vi "实验3 频率调制RX.vi"() -> ()   [LabVIEW 2015]
uses:
  <vilib>/sound2/lvsound2.llb/Sound Data Format.ctl
  <instrlib>/niUSRP/niUSRP Fetch Rx Data (CDB WDT).vi
  <vilib>/sound2/lvsound2.llb/Sound Output Write (DBL Single).vi
  <vilib>/measure/maspectr.llb/FFT Power Spectrum and PSD for 1 Chan.vi
  <vilib>/measure/NI_MAPro.lvlib
panel:
  in  "采样点数":i64=20000
  in  "天线":string(combo)="RX2"
  in  "载波频率":dbl=800000000.0 format="%#_6p"
  in  "IQ 速率":dbl=400000.0 format="%#_6p"
  in  "增益":dbl format="%#_6f"
  in  "设备IP地址":refnum<k15>="192.168.10.2"
  in  "停止":bool
  out "FM解调时域信号":waveform(dbl)(graph)={"t0"=timestamp(3578355837.194731 s since 1904-01-01), "dt"=5.000000015582913e-06, "Y"=[]}
  out "FM解调频域信号":cluster{"f0":dbl, "df":dbl, "magnitude":dbl[]}(graph)={"f0"=0.0, "df"=9.999999968834175, "magnitude"=[]}
  in  "声音格式":T1={"sample rate (S/s)"=44100.0, "number of channels"=2, "bits per sample"=16}
  # "实验3 频率调制 RX"
  # "硬件参数配置"
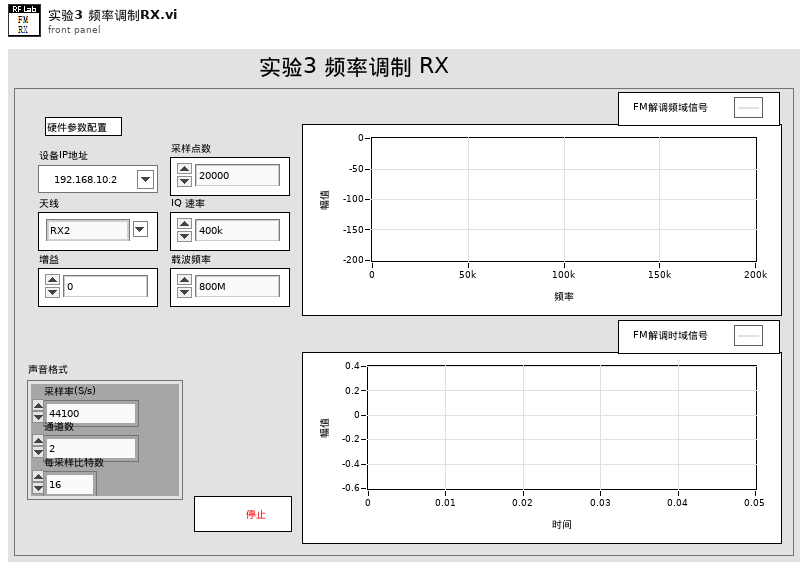
[diagram p1: front panel]
types:
  T1 = typedef "Sound Data Format.ctl" = cluster{"sample rate (S/s)":dbl, "number of channels":i32, "bits per sample":i32}
  T2 = typedef "Sound Output Task ID.ctl" = u32
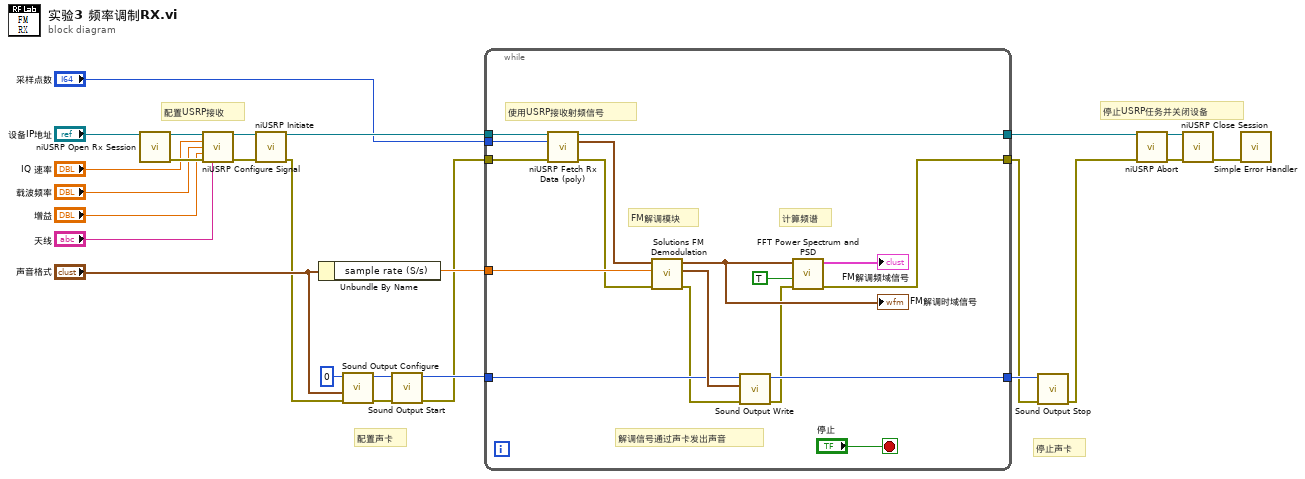
[diagram p0: block diagram]
diagram:
  # "停止USRP任务并关闭设备"
  # "配置USRP接收"
  # "停止声卡"
  # "配置声卡"
  n1 = call <instrlib>:"niUSRP Open Rx Session.vi"("device names"="设备IP地址") -> ("session handle out"=w9:refnum<k15>, "error out"=w10:errorcluster)  [unwired: 13 in]
  n2 = call <instrlib>:"niUSRP Configure Signal.vi"("session handle"=w9, "IQ rate"="IQ 速率", "carrier frequency"="载波频率", "gain"="增益", "error in (no error)"=w10, "active antenna"="天线") -> ("session handle out"=w12:refnum<k15>, "error out"=w11:errorcluster)  [unwired: 5 in, 3 out]
  n3 = call <instrlib>:"niUSRP Initiate.vi"("session handle"=w12, "error in (no error)"=w11) -> ("session handle out"=w25:refnum<k15>, "error out"=w17:errorcluster)  [unwired: 12 in]
  n4 = Unbundle By Name("声音格式") -> ("sample rate (S/s)"=w20:dbl)
  n5 = call <vilib>:"Sound Output Configure.vi"("error in (no error)"=w17, "sound format"="声音格式", "device ID"=u32 0) -> ("error out"=w22:errorcluster, "task ID"=w23:T2)  [unwired: 7 in]
  n6 = call <vilib>:"Sound Output Start.vi"("error in (no error)"=w22, "task ID"=w23) -> ("error out"=w16:errorcluster, "task ID out"=w21:T2)  [unwired: 8 in]
  n7 = while {
    tunnel: w25 -> [w43]
    tunnel: [w41] -> w26
    tunnel: "采样点数" -> [w39]
    tunnel: w21 -> [w32]
    tunnel: [w38] -> w19
    tunnel: w20 -> [w31]
    tunnel: w16 -> [w42]
    tunnel: [w27] -> w15
    stop <- "停止" stop-if-true
    # "使用USRP接收射频信号"
    # "计算频谱"
    # "解调信号通过声卡发出声音"
    # "FM解调模块"
    n8 = call-poly <instrlib>:"niUSRP Fetch Rx Data (poly).vi"("session handle"=w43, "number of samples"=w39, "error in (no error)"=w42) -> ("session handle out"=w41:refnum<k15>, "data"=w35:waveform(cdb), "error out"=w30:errorcluster)  [unwired: 9 in, 1 out]
    n9 = call "Solutions FM Demodulation.vi"("错误输入"=w30, "重采样率"=w31, "接收信号"=w35) -> ("错误输出"=w29:errorcluster, "重采样后信号"=w34:waveform(dbl), "解调后信号"=w33:waveform(dbl))  [unwired: 6 in]
    "FM解调时域信号" <- w33
    n10 = call-poly <vilib>:"Sound Output Write.vi"("error in (no error)"=w29, "data"=w34, "task ID"=w32) -> ("error out"=w28:errorcluster, "task ID out"=w38:T2)  [unwired: 7 in]
    n11 = call-poly <vilib>:"FFT Power Spectrum and PSD.vi"("error in (no error)"=w28, "dB On (F)"=TRUE, "time signal"=w33) -> ("error out"=w27:errorcluster, "Power Spectrum / PSD"=→"FM解调频域信号":cluster{"f0":dbl, "df":dbl, "magnitude":dbl[]})  [unwired: 5 in, 2 out]
  }
  n12 = call <vilib>:"Sound Output Stop.vi"("error in (no error)"=w15, "task ID"=w19) -> ("error out"=w14:errorcluster)  [unwired: 8 in, 1 out]
  n13 = call <instrlib>:"niUSRP Abort.vi"("session handle"=w26, "error in (no error)"=w14) -> ("session handle out"=w3:refnum<k15>, "error out"=w2:errorcluster)  [unwired: 12 in]
  n14 = call <instrlib>:"niUSRP Close Session.vi"("session handle"=w3, "error in (no error)"=w2) -> ("error out"=w1:errorcluster)  [unwired: 13 in]
  n15 = call <vilib>:"Simple Error Handler.vi"("error in (no error)"=w1) -> ()  [unwired: 4 in, 5 out]
